vi "hReadChannelsRTDMA2013.vi"(0 "FPGA VI Reference In":refnum<k20>, 1 "Nsamples":u32, 3 "error in":errorcluster) -> (5 "FPGA VI Reference Out":refnum<k20>, 6 "Fehler":bool, 7 "RawArray":i16[][](array[numeric]), 8 "error out":errorcluster)   [LabVIEW 2014]
doc: "startet das einlesen und führt dies bis n Samples aus\nHier mit FIFO und IRQ."
uses:
  <vilib>/Utility/error.llb/Error Cluster From Error Code.vi
  <vilib>/rvi/errors/niLvFpgaAdjustHostInterfaceError.vi
  <vilib>/RVI Host/nirviSupport.llb/nirviErrorClusterFromErrorCode.vi
  <vilib>/rvi/interface/nirviReadWriteControl/nirviReadWriteControl.xnode
  FPGA Bitfiles/W7XBolo2017_FPGATarget_FlorianDefault.lvbitx
  f_main_2014.vi
  <vilib>/rvi/interface/nirviMethod/nirviMethod.xnode
  NiFpgaLv.dll
  <vilib>/rvi/interface/nirviMethod/StockFPGA_InlinedMethodWaitForSingleIRQ.vi
  <vilib>/FPGAPlugInAG/PCI-7813R/niLvFpga_WaitOnIrq_PCI-7813R.vi
  <vilib>/FPGAPlugInAG/PCI-7813R/niLvFpga_AcknowledgeIrq_PCI-7813R.vi
  <vilib>/FPGAPlugInAG/PCI-7813R/niLvFpga_ReadFifo_PCI-7813R.vi
  <vilib>/rvi/errors/niLvFpgaMergeErrorWithErrorCode.vi
panel:
  out "STOP?":bool
  out "ScanID":u32
  out "IRQ(s) Asserted":i32
  out "Timed Out":bool
  # "Sampling"
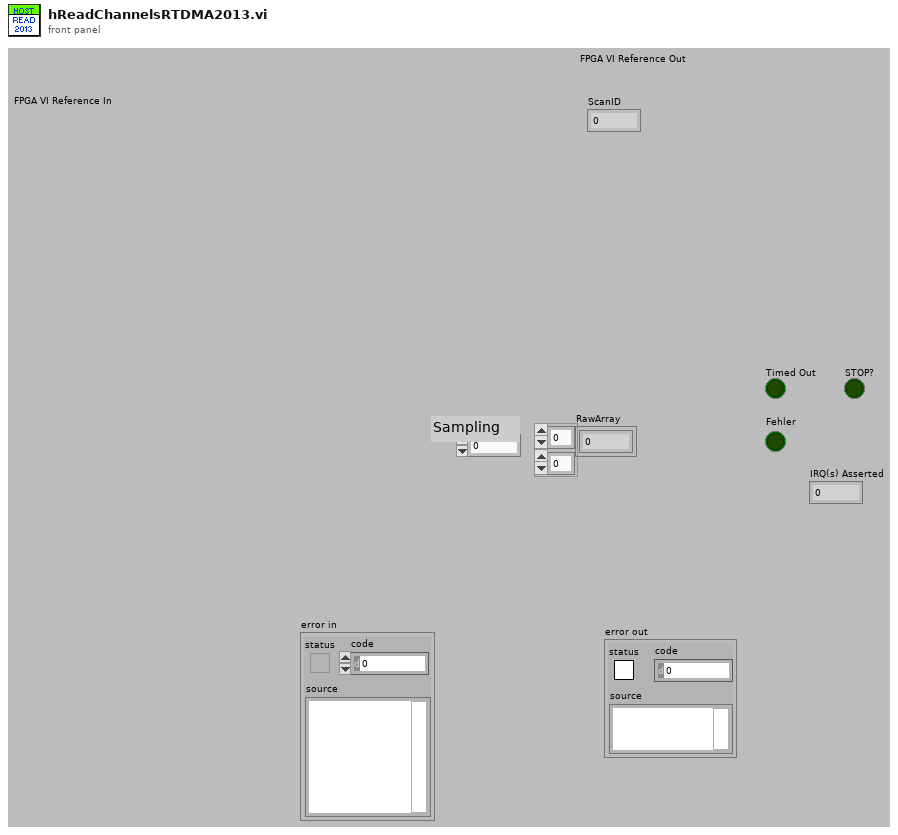
[diagram p1: front panel]
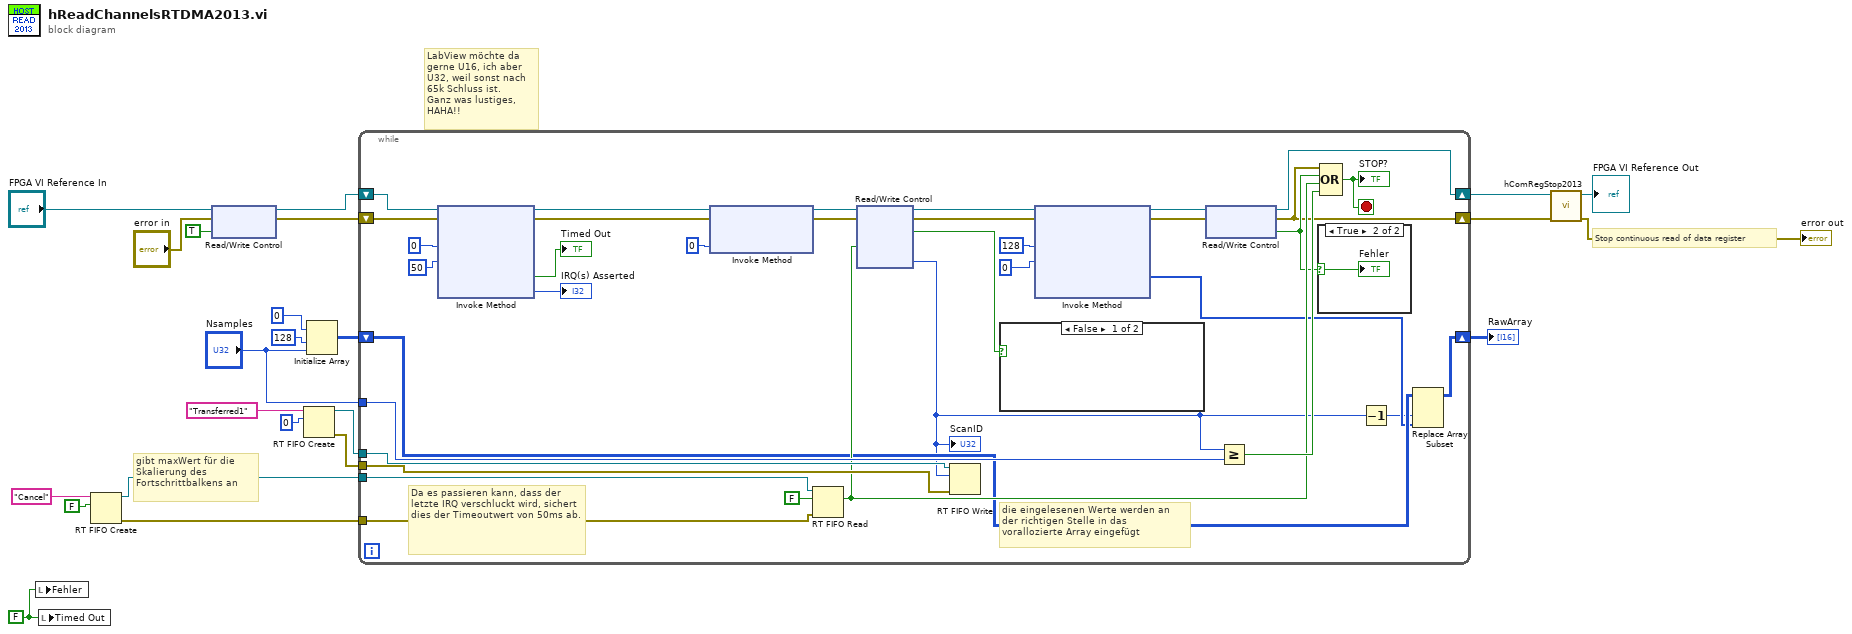
[diagram p0: block diagram]
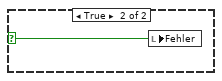
[diagram p3: hidden frame]
diagram:
  w15 = FALSE
  # "Stop continuous read of data register"
  # "gibt maxWert für die Skalierung des Fortschrittbalkens an"
  # "LabView möchte da gerne U16, ich aber U32, weil sonst nach 65k Schluss ist. \nGanz was lustiges, HAHA!!"
  n1 = local write "Fehler"(w15) -> ()
  n2 = local write "Timed Out"(w15) -> ()
  n3 = RT FIFO Create(0:"Cancel" ("name (unnamed)"), 1:FALSE) -> (8:w17:refnum<k33>, 11:w16:errorcluster)  [unwired: 2 in, 5 out]
  n4 = xnode "Read/Write Control"("FPGA VI Reference In"="FPGA VI Reference In", "error in"="error in", "ADCRead"=TRUE) -> ("FPGA VI Reference Out"=w8:refnum<k20>, "error out"=w7:errorcluster)
  n5 = RT FIFO Create(0:"Transferred1" ("name (unnamed)"), 1:u32 0) -> (8:w20:refnum<k33>, 11:w19:errorcluster)  [unwired: 2 in, 5 out]
  n6 = Initialize Array(i16 0, 128 ("dimension size"), "Nsamples") -> (w23:i16[][])
  n7 = while {
    tunnel: "Nsamples" -> [w46]
    shift-right: [w47] -> w12
    shift-left: w23 -> [w33]
    shift-right: [w54] -> w4
    shift-left: w8 -> [w57]
    shift-right: [w24] -> w6
    shift-left: w7 -> [w56]
    tunnel: w20 -> [w44]
    tunnel: w19 -> [w43]
    tunnel: w17 -> [w41]
    tunnel: w16 -> [w40]
    stop <- w45 stop-if-true
    # "die eingelesenen Werte werden an der richtigen Stelle in das vorallozierte Array eingefügt"
    # "Da es passieren kann, dass der letzte IRQ verschluckt wird, sichert dies der Timeoutwert von 50ms ab."
    n8 = xnode "Invoke Method"("FPGA VI Reference In"=w57, "error in"=w56, "IRQ Number(s)"=0, "Timeout (ms)"=50) -> ("FPGA VI Reference Out"=w53:refnum<k20>, "error out"=w52:errorcluster, "Timed Out"=→"Timed Out":bool, "IRQ(s) Asserted"=→"IRQ(s) Asserted":i32)
    n9 = xnode "Invoke Method"("FPGA VI Reference In"=w53, "error in"=w52, "IRQ Number(s)"=0 ("IRQ Number")) -> ("FPGA VI Reference Out"=w50:refnum<k20>, "error out"=w49:errorcluster)
    n10 = RT FIFO Read(0:w41, 1:FALSE ("element"), 3:w40) -> (9:w42:bool)  [unwired: 5 out]
    n11 = xnode "Read/Write Control"("FPGA VI Reference In"=w50, "error in"=w49, "cancel"=w42) -> ("FPGA VI Reference Out"=w35:refnum<k20>, "error out"=w34:errorcluster, "Timeout"=w38:bool, "ScanID"=w29:u32)
    "ScanID" <- w29
    n12 = RT FIFO Write(0:w44, 1:w29, 3:w43) -> ()  [unwired: 1 in, 5 out]
    n13 = case shown="False" w38 {
      selector: w38 -> [_ w60]
      frame False {
      }
      frame True {
        n14 = local write "Fehler"(w60) -> ()
      }
    }
    n15 = xnode ("Invoke Method")("FPGA VI Reference In"=w35, "error in"=w34, "Number of Elements"=u32 128, "Timeout (ms)"=0 ("Timeout")) -> ("FPGA VI Reference Out"=w27:refnum<k20>, "error out"=w26:errorcluster, "Data"=w32:u32[])  [unwired: 1 out]
    n16 = xnode "Read/Write Control"("FPGA VI Reference In"=w27, "error in"=w26) -> ("FPGA VI Reference Out"=w54:refnum<k20>, "error out"=w24:errorcluster, "Fifo-Fehler"=w25:bool)
    n17 = Greater Or Equal?(x=w29, y=w46) -> (x >= y?=w58:bool)
    n18 = case shown="True" w25 {
      selector: w25 -> [_ w59]
      frame False {
      }
      frame True {
        "Fehler" <- w59
      }
    }
    n19 = Compound Arithmetic op=OR(w24, w25, w42, w58) -> (w45:bool)
    "STOP?" <- w45
    n20 = Decrement(x=w29) -> (x-1=w28:u32)
    n21 = Replace Array Subset(array=w33, new element=w32, index (col)=w28) -> (w47:i16[][])  [unwired: 1 in]
  }
  "RawArray" <- w12
  n22 = call "hComRegStop2013.vi"("error in"=w6, "FPGA VI Reference In"=w4) -> ("error out"=→"error out":errorcluster, "FPGA VI Reference Out"=→"FPGA VI Reference Out":refnum<k20>)  [unwired: 3 in, 1 out]
